vi "Lights Controller.vi"(8 "error in":errorcluster) -> ()   [LabVIEW 2020]
doc: "This VI executes continuously carrying out the current operation and responding to updates or new operations. It will often contain the timing or control code that is difficult to place directly in TeleOp. This VI generally opens all sensors and motors and isolates the rest of the robot code from knowing how the operations are carried out."
uses:
  <vilib>/Rock Robotics/WPI/Framework/Completion Status.ctl
  Lights Setpoints.ctl
  Lights Operations.ctl
  <vilib>/Rock Robotics/SystemInterfaces/DIO/FPGA_DIOPWMChannel.ctl
  Framework/Robot Global Data.vi
  source files/ArduinoSerialBling.lvlib
  <vilib>/Rock Robotics/Network Tables/NT Write Boolean.vi
panel:
  out "size(s)":i32
  in  "Pit Sin Rate":i32=100
  in  "White":u32(colorbox)=16747144
  in  "Blending LEDs":u8=10
  in  "String Length":u16=100
  in  "Interactive Values":T1
  out "Current\nCmd":string
  in  "Buttons":cluster{"Execute Cmd":bool, "Abort Cmd":bool}
  out "Command Timing":cluster{"Start Time (ms)":u32, "Iterations":i32}
  out "Status":T3
  # "Tip: It may be helpful to observe inputs and sensor values.\nYou may also want to display tuning or debugging controls."
  # "should be 20"
  # "Interactive Command: You may fill in the settings for a command\nand schedule it with the Execute button. You can observe and abort\nany command while fine tuning the code for the controller."
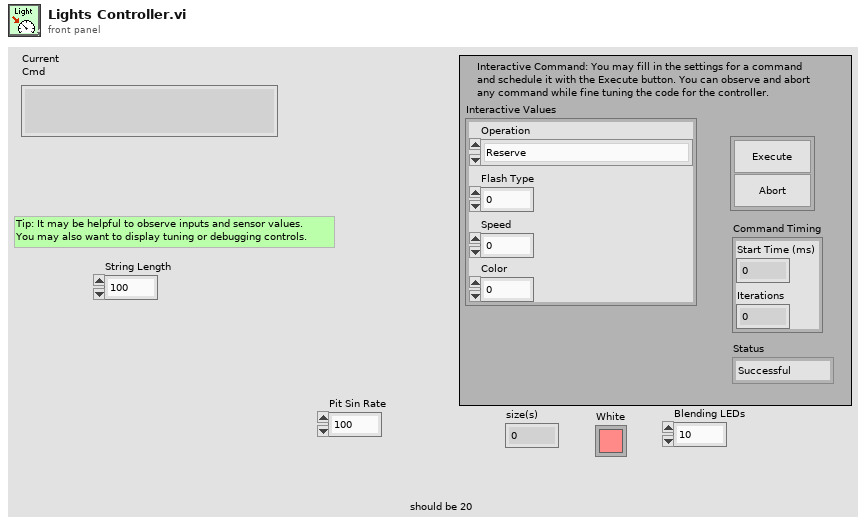
[diagram p1: front panel]
types:
  T1 = typedef "Lights Setpoints.ctl" = cluster{"Operation":T2, "Color":dbl, "Flash Type":dbl, "Speed":dbl}
  T2 = typedef "Lights Operations.ctl" = enum16{"Reserve", "Read Current", "Immediate"}
  T3 = typedef "Completion Status.ctl" = enum16{"Successful", "Aborted", "Incomplete"}
  T4 = typedef "FPGA_DIOPWMChannel.ctl" = enum8{"PWM 0", "PWM 1", "PWM 2", "PWM 3", "PWM 4", "PWM 5", "PWM 6", "PWM 7", "PWM 8", "PWM 9", "PWM MXP 0", "PWM MXP 1", "PWM MXP 2", "PWM MXP 3", "PWM MXP 4", "PWM MXP 5", "PWM MXP 6", "PWM MXP 7", "PWM MXP 8", "PWM MXP 9", "Invalid"}
  T5 = typedef "WPI_PWMDeviceRef.ctl" = cluster{"DeviceStatus":errorcluster, "PWM Channel":T4}
  T6 = typedef "Command Status Info.ctl" = cluster{"Name":string, "Status":T3, "notifier out":T7}
  T7 = typedef "Completion Notifier.ctl" = refnum<notifier>
  T8 = cluster{"Current Command":T1, "Command Timing":cluster{"Start Time (ms)":u32, "Iterations":i32}, "Command Arguments":cluster{"Command Info":T6, "Description":string, "Default Command":T1, "queue out":refnum<queue>, "Subsystem Name":string}}
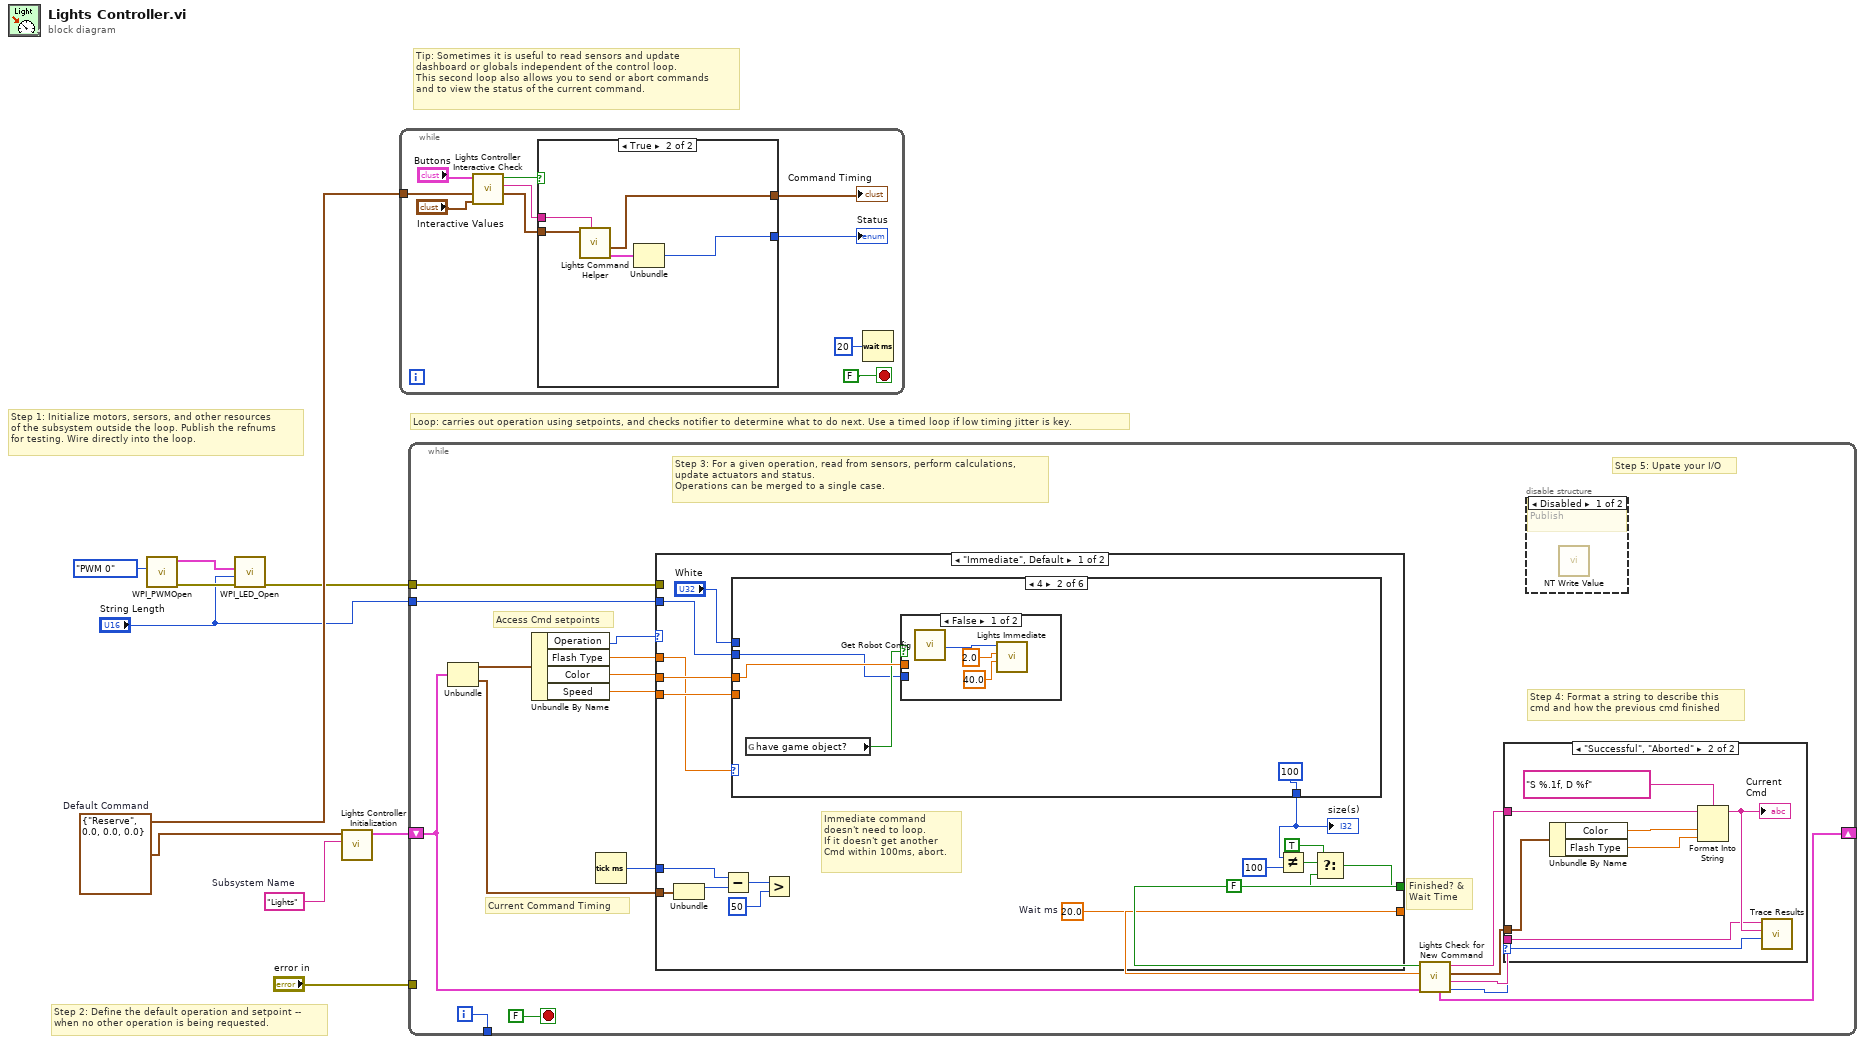
[diagram p0: block diagram]
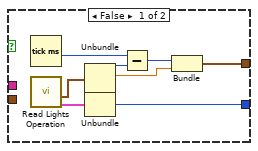
[diagram p2: hidden frame]
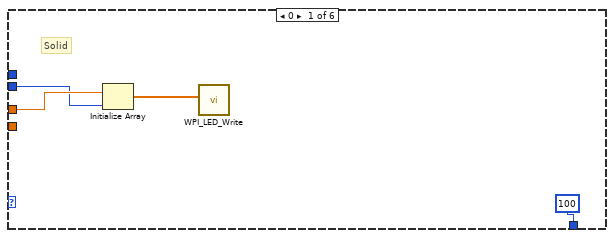
[diagram p5: hidden frame]
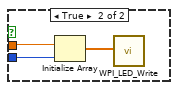
[diagram p6: hidden frame]
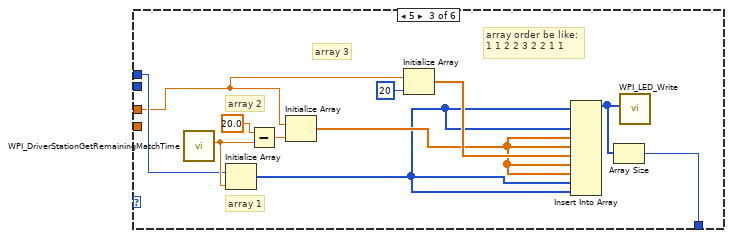
[diagram p7: hidden frame]
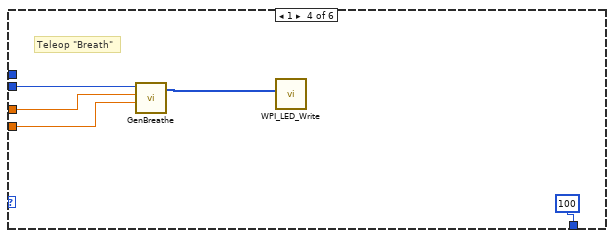
[diagram p8: hidden frame]
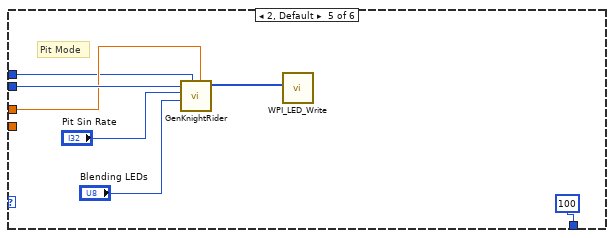
[diagram p9: hidden frame]
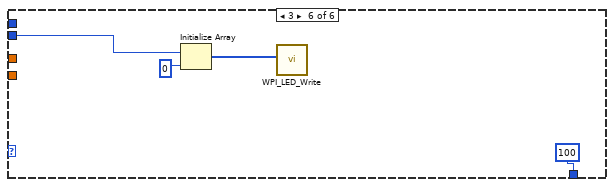
[diagram p10: hidden frame]
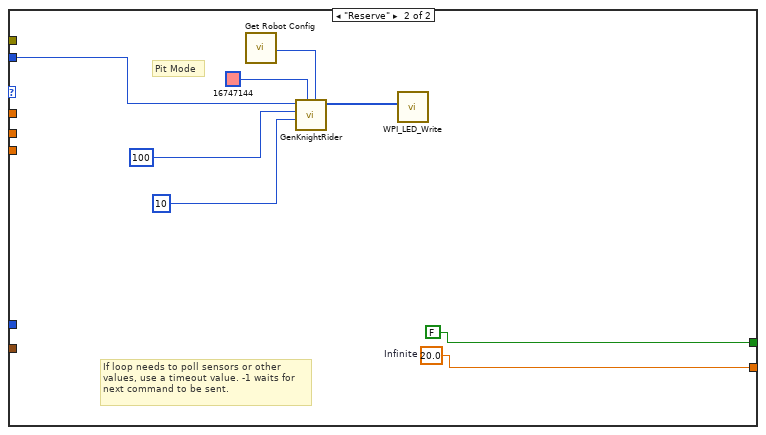
[diagram p11: hidden frame]
diagram:
  w6 = T1 {"Operation"=enum."Reserve", "Color"=0.0, "Flash Type"=0.0, "Speed"=0.0}  # Default Command
  w7 = "Lights"  # Subsystem Name
  # "Tip: Sometimes it is useful to read sensors and update\ndashboard or globals independent of the control loop.\nThis second loop also allows you to send or abort commands\nand to view the status of the current command."
  # "Step 2: Define the default operation and setpoint --\nwhen no other operation is being requested."
  # "Step 1: Initialize motors, sersors, and other resources\nof the subsystem outside the loop. Publish the refnums\nfor testing. Wire directly into the loop."
  # "Loop: carries out operation using setpoints, and checks notifier to determine what to do next. Use a timed loop if low timing jitter is key."
  n1 = call <vilib>:"WPI_PWMOpen.vi"("PWM Channel"=FPGA_DIOPWMChannel."PWM 0") -> ("error out"=w4:errorcluster, "PWMDeviceRef"=w5:T5)  [unwired: 9 in]
  n2 = call <vilib>:"WPI_LED_Open.vi"("error in"=w4, "String Length"="String Length", "PWMDeviceRef"=w5) -> ("error out"=w2:errorcluster)  [unwired: 8 in]
  n3 = call "Lights Controller Initialization.vi"("Subsystem Name"=w7, "Default Command"=w6) -> ("Current Command"=w8:T8)  [unwired: 9 in]
  n4 = while {
    tunnel: w6 -> [w16]
    stop <- FALSE stop-if-true
    n5 = call "Lights Controller Interactive Check.vi"("Interactive Command in"="Interactive Values", "Default Command"=w16, "Buttons"="Buttons") -> ("Interactive Command out"=w13:T1, "Trace String"=w14:string, "Schedule"=w15:bool)  [unwired: 6 in]
    n6 = case shown="True" w15 {
      tunnel: [w27 w32] -> w12
      tunnel: w13 -> [_ w30]
      tunnel: [w23 w28] -> w11
      tunnel: w14 -> [_ w31]
      frame False {
        n7 = Tick Count (ms)() -> (millisecond timer value=w22:u32)
        n8 = call "Read Lights Operation.vi"() -> ("Command Info"=w20:T6, "SubSystem Data"=w21:T1)  [unwired: 9 in, 1 out]
        n9 = Unbundle(w21) -> ("Operation"=w26:T2, "Color"=w24:dbl)  [unwired: 2 out]
        n10 = Unbundle(w20) -> ("Status"=w27:T3)  [unwired: 2 out]
        n11 = Subtract(x=w22, y=w26) -> (x-y=w25:u32)
        n12 = Bundle(w25, "Color"=w24) -> (w23:cluster{u32, "Color":dbl})  [unwired: 1 in]
      }
      frame True {
        n13 = call "Lights Command Helper.vi"("Description"=w31, "SubSystem Data"=w30) -> ("Command Info Out"=w29:T6, "Command Timing"=w28:cluster{"Start Time (ms)":u32, "Iterations":i32})  [unwired: 7 in, 1 out]
        n14 = Unbundle(w29) -> ("Status"=w32:T3)  [unwired: 2 out]
      }
    }
    "Status" <- w12
    "Command Timing" <- w11
    n15 = Wait (ms)(milliseconds to wait=u32 20) -> ()  [unwired: 1 out]
  }
  n16 = while {
    shift-right: [w43] -> _
    shift-left: w8 -> [w36]
    tunnel: [w50] -> _
    tunnel: "error in" -> [_]
    tunnel: w2 -> [w34]
    tunnel: "String Length" -> [w33]
    i -> [w50]
    stop <- FALSE stop-if-true
    # "Step 5: Upate your I/O"
    # "Step 4: Format a string to describe this\ncmd and how the previous cmd finished"
    # "Current Command Timing"
    # "Access Cmd setpoints"
    # "Finished? &\nWait Time"
    # "Step 3: For a given operation, read from sensors, perform calculations,\nupdate actuators and status.\nOperations can be merged to a single case."
    n17 = Unbundle(w36) -> ("Current Command"=w49:T1, "Command Timing"=w45:cluster{"Start Time (ms)":u32, "Iterations":i32})  [unwired: 1 out]
    n18 = Unbundle By Name(w49) -> ("Operation"=w48:T2, "Flash Type"=w47:dbl, "Color"=w44:dbl, "Speed"=w35:dbl)
    n19 = Tick Count (ms)() -> (millisecond timer value=w46:u32)
    n20 = case shown="\"Immediate\", Default" w48 {
      tunnel: [w76 w125] -> w41
      tunnel: [w61 FALSE ("ignore previous (F)")] -> w42
      tunnel: w45 -> [w72 _]
      tunnel: w47 -> [w67 _]
      tunnel: w46 -> [w71 _]
      tunnel: w44 -> [w69 _]
      tunnel: w35 -> [w68 _]
      tunnel: w34 -> [_ _]
      tunnel: w33 -> [w70 w120]
      frame "Immediate", Default {
        w76 = 20.0  # Wait ms
        # "Immediate command\ndoesn't need to loop.\nIf it doesn't get another\nCmd within 100ms, abort."
        n21 = Unbundle(w72) -> ("Start Time (ms)"=w75:u32)  [unwired: 1 out]
        n22 = Subtract(x=w71, y=w75) -> (x-y=w74:u32)
        n23 = case shown="4" w67 {
          tunnel: w70 -> [w78 w82 _ w103 w111 w115]
          tunnel: w69 -> [w79 w84 w94 w104 w109 _]
          tunnel: w68 -> [_ _ _ w105 _ _]
          tunnel: "White" -> [_ _ w99 _ w108 _]
          tunnel: [100 100 w91 100 100 100] -> w64
          frame 0 {
            # "Solid"
            n24 = Initialize Array(w79, w78) -> (w80:dbl[])
            n25 = call <vilib>:"WPI_LED_Write.vi"("Color Array"=w80) -> ()  [unwired: 10 in, 1 out]
          }
          frame 4 {
            n26 = global read "Robot Global Data.vi" "have game object?"() -> (w83:bool)
            n27 = case shown="False" w83 {
              tunnel: w84 -> [_ w90]
              tunnel: w82 -> [_ w88]
              frame False {
                n28 = call "Get Robot Config.vi"() -> ("Color"=w85:u32)  [unwired: 12 in, 7 out]
                n29 = call "Lights Immediate.vi"("Speed"=40.0, "Flash Type"=2.0, "Color"=w85) -> ()  [unwired: 8 in, 1 out]
              }
              frame True {
                n30 = Initialize Array(w90, w88) -> (w89:dbl[])
                n31 = call <vilib>:"WPI_LED_Write.vi"("Color Array"=w89) -> ()  [unwired: 10 in, 1 out]
              }
            }
          }
          frame 5 {
            # "array order be like:\n1 1 2 2 3 2 2 1 1"
            # "array 1"
            # "array 2"
            # "array 3"
            n32 = call <vilib>:"WPI_DriverStationGetRemainingMatchTime.vi"() -> ("Match Time(s)"=w100:sgl)  [unwired: 10 in, 1 out]
            n33 = Initialize Array(w99, w100) -> (w95:u32[])
            n34 = Subtract(x=sgl 20.0, y=w100) -> (x-y=w101:sgl)
            n35 = Initialize Array(w94, w101) -> (w96:dbl[])
            n36 = Initialize Array(w94, 20 ("dimension size")) -> (w97:dbl[])
            n37 = Insert Into Array(array=w95, new element #1=w95, new element #2=w96, new element #3=w96, new element #4=w97, new element #5=w96, new element #6=w96, new element #7=w95, new element #8=w95) -> (w93:u32[])  [unwired: 1 in]
            n38 = Array Size(array=w93) -> (size(s)=w91:i32)
            n39 = call <vilib>:"WPI_LED_Write.vi"("Color Array"=w93) -> ()  [unwired: 10 in, 1 out]
          }
          frame 1 {
            # "Teleop \"Breath\""
            n40 = call "GenBreathe.vi"("Sine Rate"=w105, "Color Box"=w104, "NumLeds"=w103) -> ("Array"=w106:u32[])  [unwired: 7 in, 1 out]
            n41 = call <vilib>:"WPI_LED_Write.vi"("Color Array"=w106) -> ()  [unwired: 10 in, 1 out]
          }
          frame 2, Default {
            # "Pit Mode"
            n42 = call "GenKnightRider.vi"("Background Color"=w109, "Foreground Color"=w108, "Blending LEDs"="Blending LEDs", "Sine Rate"="Pit Sin Rate", "NumLeds"=w111) -> ("Array"=w110:u32[])  [unwired: 5 in, 1 out]
            n43 = call <vilib>:"WPI_LED_Write.vi"("Color Array"=w110) -> ()  [unwired: 10 in, 1 out]
          }
          frame 3 {
            n44 = Initialize Array(w115, 0 ("dimension size")) -> (w117:u16[])
            n45 = call <vilib>:"WPI_LED_Write.vi"("Color Array"=w117) -> ()  [unwired: 10 in, 1 out]
          }
        }
        "size(s)" <- w64
        n46 = Greater?(x=w74, y=u8 50 ("Left Motor")) -> ()  [unwired: 1 out]
        n47 = Not Equal?(x=w64, y=100) -> (x != y?=w65:bool)
        n48 = Select(t=TRUE, s=w65, f=FALSE ("ignore previous (F)")) -> (s? t:f=w61:bool)
      }
      frame "Reserve" {
        w125 = 20.0  # Infinite
        # "Pit Mode"
        # "If loop needs to poll sensors or other\nvalues, use a timeout value. -1 waits for\nnext command to be sent."
        n49 = call "Get Robot Config.vi"() -> ("Color"=w118:u32)  [unwired: 12 in, 7 out]
        n50 = call "GenKnightRider.vi"("Background Color"=w118, "Foreground Color"=u32 16747144 ("White 2"), "Blending LEDs"=u8 10 ("Blending LEDs 2"), "Sine Rate"=100 ("Pit Sin Rate 2"), "NumLeds"=w120) -> ("Array"=w123:u32[])  [unwired: 5 in, 1 out]
        n51 = call <vilib>:"WPI_LED_Write.vi"("Color Array"=w123) -> ()  [unwired: 10 in, 1 out]
      }
    }
    n52 = call "Lights Check for New Command.vi"("Current Command"=w36, "Wait time (ms)"=w41, "Finished?"=w42) -> ("Completion"=w37:T3, "Subsystem Name"=w38:string, "Current Command"=w39:T1, "Initial Trace String"=w40:string, "NextCommand"=w43:T8)  [unwired: 4 in]
    n53 = case shown="\"Successful\", \"Aborted\"" w37 {
      selector: w37 -> [_ w59]
      tunnel: w40 -> [_ w55]
      tunnel: w39 -> [_ w56]
      tunnel: w38 -> [_ w52]
      frame "Incomplete", Default {
        # "Continuing current command"
      }
      frame "Successful", "Aborted" {
        # "Report and setup for next command"
        n54 = Unbundle By Name(w56) -> ("Color"=w58:dbl, "Flash Type"=w53:dbl)
        n55 = Format Into String(format string="S %.1f, D %f", initial string=w55, w58, w53) -> (resulting string=w54:string)  [unwired: 1 in, 1 out]
        "Current\nCmd" <- w54
        n56 = call <vilib>:"Trace Results.vi"("Status of previous command"=w59, "Description"=w54, "Subsystem"=w52) -> ()  [unwired: 9 in]
      }
    }
    n57 = disable-structure shown="Disabled" {
      frame Disabled {
        # "Publish"
        n58 = call-poly <vilib>:"NT Write Value.vi"() -> ()  [unwired: 11 in, 1 out]
      }
      frame Enabled {
      }
    }
  }
